vi "SetParam.vi"(8 "error in (no error)":errorcluster caption="entrée d'erreur (pas d'erreur)", 10 "multilabel_confusion_matrix":T1={"sample_weight"=[], "labels"={"dtype_labels"="None", "labels"=["None"]}, "samplewise"=FALSE}, 11 "Multilabel_Confusion_Matrix.lvclass":refnum<class "Multilabel_Confusion_Matrix.lvclass">) -> (0 "error out":errorcluster caption="sortie d'erreur", 3 "Multilabel_Confusion_Matrix.lvclass":refnum<class "Multilabel_Confusion_Matrix.lvclass">)   [LabVIEW 2020, in "Multilabel_Confusion_Matrix.lvclass"]
doc: "Set Parameters"
uses:
  Multilabel_Confusion_Matrix.lvclass
  Multilabel_Confusion_Matrix.lvclass/Multilabel_Confusion_Matrix.ctl
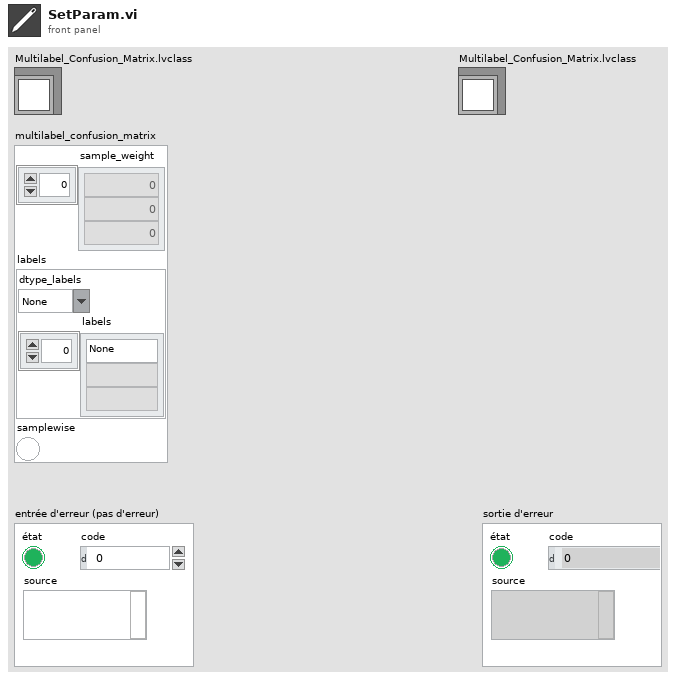
[diagram p1: front panel]
types:
  T1 = cluster{"sample_weight":dbl[], "labels":cluster{"dtype_labels":string, "labels":string[]}, "samplewise":bool}
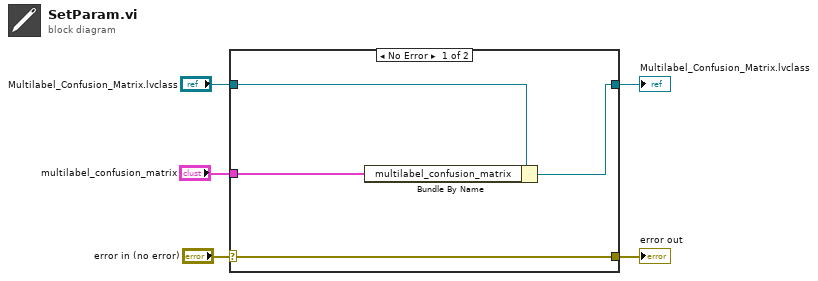
[diagram p0: block diagram]
diagram:
  n1 = case shown="No Error" "error in (no error)" {
    selector: "error in (no error)" -> [w9 w10]
    tunnel: [w9 w10] -> w4
    tunnel: [w7 w11] -> w2
    tunnel: "Multilabel_Confusion_Matrix.lvclass" -> [w8 w11]
    tunnel: "multilabel_confusion_matrix" -> [w6 _]
    frame No Error {
      n2 = Bundle By Name(cluster=w8, "multilabel_confusion_matrix"=w6) -> (w7:refnum<class "Multilabel_Confusion_Matrix.lvclass">)
    }
    frame Error {
    }
  }
  "error out" <- w4
  "Multilabel_Confusion_Matrix.lvclass" <- w2
